vi "OS Title Bar Compatibility.vi"(9 "Upper Splitter":refnum<vi>, 10 "Title Panel":refnum<vi>, 11 "VI in":refnum<vi>) -> (0 "error out":errorcluster)   [LabVIEW 2019, in "Panther Dashboard.lvlib"]
uses:
  Panther Dashboard.lvlib
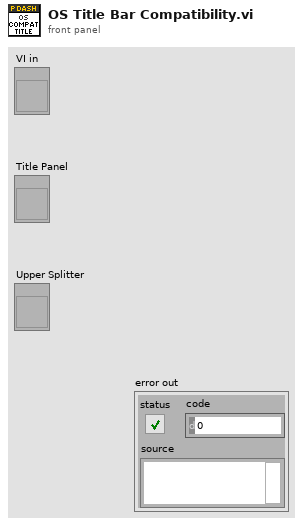
[diagram p1: front panel]
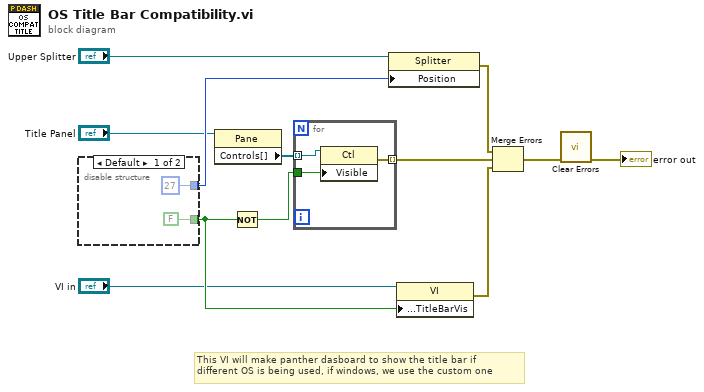
[diagram p0: block diagram]
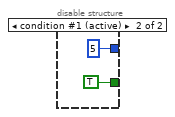
[diagram p2: hidden frame]
diagram:
  # "This VI will make panther dasboard to show the title bar if\ndifferent OS is being used, if windows, we use the custom one"
  n1 = disable-structure shown="Default" {
    disable-tunnel: [FALSE TRUE] -> w7
    disable-tunnel: [27 ("Splitter Position") 5 ("Splitter Position")] -> w8
    frame condition #0 {
    }
    frame condition #1 (active) {
    }
  }
  n2 = property class="Pane"(reference="Title Panel") -> ("Controls[]"=w4:refnum<vi>[])  [unwired: 1 in, 2 out]
  n3 = Not(x=w7) -> (.not. x?=w5:bool)
  n4 = for {
    tunnel: w4 -> [w18] mode=indexing
    tunnel: w5 -> [w17]
    tunnel: [w19] -> w1 mode=indexing
    n5 = property class="Ctl"(reference=w18, "Visible"=w17) -> (error out=w19:errorcluster)  [unwired: 1 in, 1 out]
  }
  n6 = property class="Splitter"(reference="Upper Splitter", "Position"=w8) -> (error out=w12:errorcluster)  [unwired: 1 in, 1 out]
  n7 = property class="VI"(reference="VI in", "Front Panel.TitleBarVis"=w7) -> (error out=w11:errorcluster)  [unwired: 1 in, 1 out]
  n8 = Merge Errors(w12, w1, w11) -> (w10:errorcluster)
  n9 = call <vilib>:"Clear Errors.vi"("error in (no error)"=w10) -> ("error out"=→"error out":errorcluster)  [unwired: 5 in, 1 out]
